vi "Build Chamber State Payload.vi"(8 "error in (no error)":errorcluster, 11 "Thermal Chamber Controller In":refnum<class "Thermal Chamber Controller.lvclass">) -> (0 "error out":errorcluster, 2 "Chamber Status Reply Payload":T1={"Actual Temperature"=0.0, "Temperature Set Point"=0.0, "Temperature Ramp Rate"=0.0, "Heater State"=enum."Heater Enabled"}, 3 "Thermal Chamber Controller Out":refnum<class "Thermal Chamber Controller.lvclass">)   [LabVIEW 2020, in "Thermal Chamber Controller.lvclass"]
uses:
  Thermal Chamber Controller.lvclass
  Private/Heater State.ctl
  Public/Chamber State.ctl
  Thermal Chamber Response Simlator/Thermal Chamber Response Simlator.lvclass
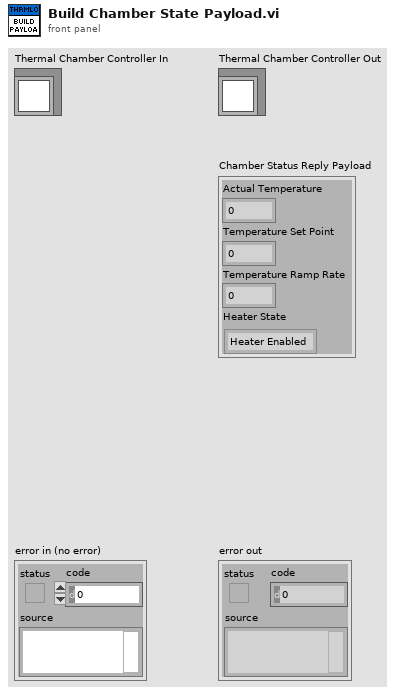
[diagram p1: front panel]
types:
  T1 = typedef "Thermal Chamber Controller.lvclass/Chamber State.ctl" = cluster{"Actual Temperature":dbl, "Temperature Set Point":dbl, "Temperature Ramp Rate":dbl, "Heater State":T2}
  T2 = typedef "Thermal Chamber Controller.lvclass/Heater State.ctl" = enum16{"Heater Disabled", "Heater Enabled"}
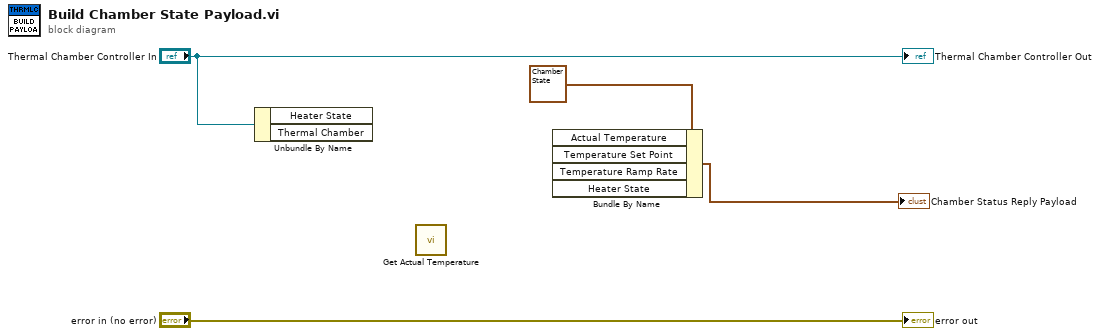
[diagram p0: block diagram]
diagram:
  n1 = Unbundle By Name("Thermal Chamber Controller In") -> ()  [unwired: 2 out]
  n2 = call "Get Actual Temperature.vi"() -> ()  [unwired: 9 in, 3 out]
  n3 = Bundle By Name(cluster=T1 {"Actual Temperature"=0.0, "Temperature Set Point"=0.0, "Temperature Ramp Rate"=0.0, "Heater State"=enum."Heater Enabled"} ("Chamber Status Reply Payload")) -> (→"Chamber Status Reply Payload":T1)  [unwired: 4 in]
  "error out" <- "error in (no error)"
  "Thermal Chamber Controller Out" <- "Thermal Chamber Controller In"
